vi "JH setpoint feedback off before point spectra.vi"() -> ()   [LabVIEW 2014]
uses:
  <userlib>/Nanonis Prog Interface V5/Nanonis Prog Interface.lvlib
panel:
  in  "spectroscopy feedback setpoint (V)":sgl=0.1 format="%_5p"
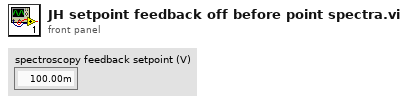
[diagram p1: front panel]
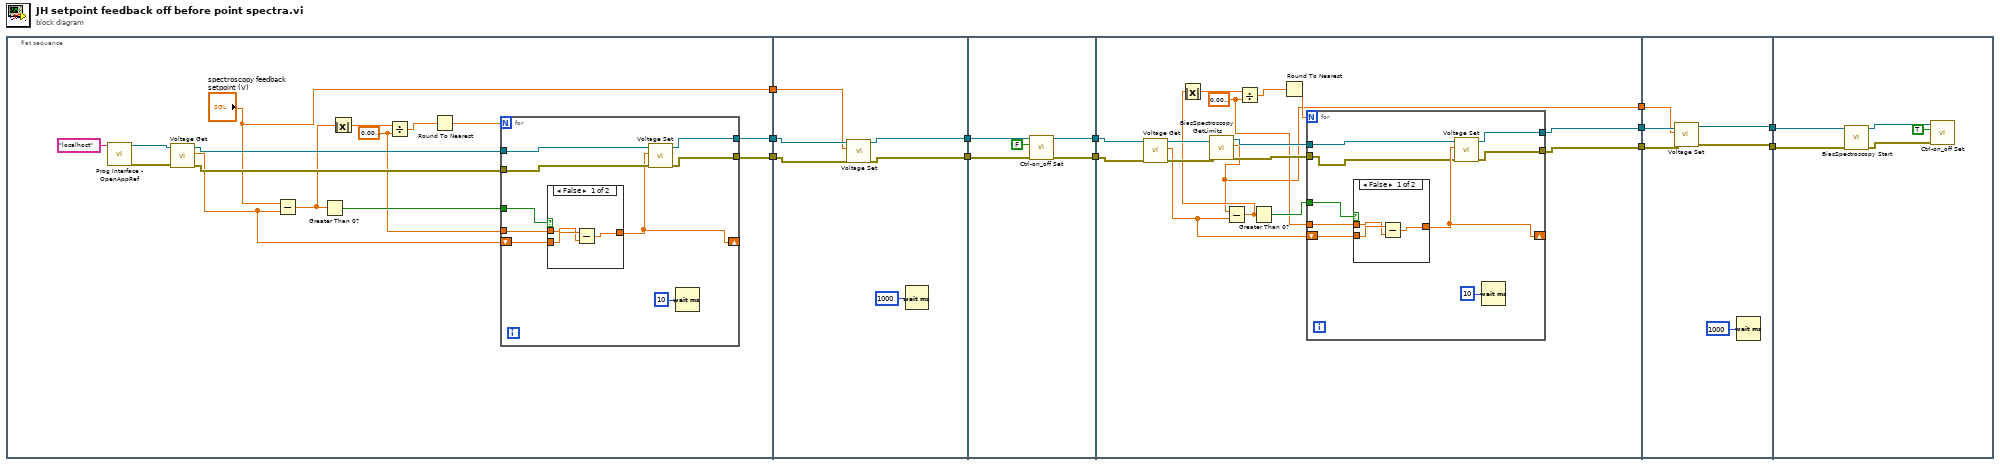
[diagram p0: block diagram]
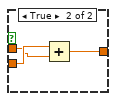
[diagram p2: hidden frame]
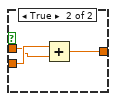
[diagram p3: hidden frame]
diagram:
  n1 = flat-sequence {
    tunnel: [w15] -> w4
    tunnel: [w14] -> w3
    tunnel: ["spectroscopy feedback setpoint (V)"] -> w2
    tunnel: [w45] -> w12
    tunnel: [w44] -> w11
    tunnel: w3 -> [w46]
    tunnel: w4 -> [w47]
    tunnel: w2 -> [w43]
    tunnel: w12 -> [w53]
    tunnel: w11 -> [w52]
    tunnel: [w50] -> w10
    tunnel: [w49] -> w9
    tunnel: w10 -> [w67]
    tunnel: w9 -> [w65]
    tunnel: [w56] -> w8
    tunnel: [w55] -> w6
    tunnel: [w54] -> w1
    tunnel: w8 -> [w89]
    tunnel: [w87] -> w7
    tunnel: w6 -> [w88]
    tunnel: [w86] -> w5
    tunnel: w1 -> [w85]
    tunnel: w7 -> [w95]
    tunnel: w5 -> [w94]
    frame #0 {
      w16 = sgl 0.01 ("y")
      n2 = call <userlib>:"Prog Interface - OpenAppRef.vi"("Machine name (local machine IP)"="localhost") -> ("Error out"=w25:errorcluster, "Application reference"=w26:refnum<vi>)  [unwired: 5 in]
      n3 = call <userlib>:"Voltage Get.vi"("error in (no error)"=w25, "Application ref in"=w26) -> ("error out"=w23:errorcluster, "Bias (V)"=w17:sgl, "Application ref out"=w24:refnum<vi>)  [unwired: 7 in]
      n4 = Subtract(x="spectroscopy feedback setpoint (V)", y=w17) -> (x-y=w21:sgl)
      n5 = Greater Than 0?(x=w21) -> (x > 0?=w22:bool)
      n6 = Absolute Value(x=w21) -> (abs(x)=w20:sgl)
      n7 = Divide(x=w20, y=w16) -> (x/y=w19:sgl)
      n8 = Round To Nearest(number=w19) -> (nearest integer value=w18:sgl)
      n9 = for {
        N: w18 -> [_]
        tunnel: w24 -> [w36]
        tunnel: w23 -> [w35]
        tunnel: w22 -> [w34]
        tunnel: w16 -> [w33]
        shift-right: [w31] -> _
        shift-left: w17 -> [w32]
        tunnel: [w29] -> w15
        tunnel: [w28] -> w14
        n10 = case shown="False" w34 {
          tunnel: w33 -> [w38 w41]
          tunnel: w32 -> [w39 w42]
          tunnel: [w37 w40] -> w31
          frame False {
            n11 = Subtract(x=w39, y=w38) -> (x-y=w37:sgl)
          }
          frame True {
            n12 = Add(x=w42, y=w41) -> (x+y=w40:sgl)
          }
        }
        n13 = call <userlib>:"Voltage Set.vi"("Error in (no error)"=w35, "Bias (V)"=w31, "Application ref in"=w36) -> ("Error out"=w28:errorcluster, "Application ref out"=w29:refnum<vi>)  [unwired: 7 in]
        n14 = Wait (ms)(milliseconds to wait=u32 10) -> ()  [unwired: 1 out]
      }
    }
    frame #1 {
      n15 = call <userlib>:"Voltage Set.vi"("Error in (no error)"=w46, "Bias (V)"=w43, "Application ref in"=w47) -> ("Error out"=w44:errorcluster, "Application ref out"=w45:refnum<vi>)  [unwired: 7 in]
      n16 = Wait (ms)(milliseconds to wait=u32 1000) -> ()  [unwired: 1 out]
    }
    frame #2 {
      n17 = call <userlib>:"Ctrl-on_off Set.vi"("error in (no error)"=w52, "Z Controller ON/OFF"=FALSE, "Application ref in"=w53) -> ("error out"=w49:errorcluster, "Application ref out"=w50:refnum<vi>)  [unwired: 7 in]
    }
    frame #3 {
      w57 = sgl 0.01 ("y")
      n18 = call <userlib>:"Voltage Get.vi"("error in (no error)"=w65, "Application ref in"=w67) -> ("error out"=w64:errorcluster, "Bias (V)"=w62:sgl, "Application ref out"=w66:refnum<vi>)  [unwired: 7 in]
      n19 = call <userlib>:"BiasSpectroscopy GetLimits.vi"("Error in (no error)"=w64, "Application ref in"=w66) -> ("Error out"=w68:errorcluster, "Start value (V)"=w54:sgl, "Application ref out"=w69:refnum<vi>)  [unwired: 4 in, 1 out]
      n20 = Subtract(x=w54, y=w62) -> (x-y=w58:sgl)
      n21 = Absolute Value(x=w58) -> (abs(x)=w61:sgl)
      n22 = Divide(x=w61, y=w57) -> (x/y=w60:sgl)
      n23 = Greater Than 0?(x=w58) -> (x > 0?=w63:bool)
      n24 = Round To Nearest(number=w60) -> (nearest integer value=w59:sgl)
      n25 = for {
        N: w59 -> [_]
        tunnel: w69 -> [w71]
        tunnel: w63 -> [w78]
        tunnel: w57 -> [w77]
        shift-right: [w75] -> _
        shift-left: w62 -> [w76]
        tunnel: [w73] -> w56
        tunnel: [w72] -> w55
        tunnel: w68 -> [w70]
        n26 = case shown="False" w78 {
          tunnel: w77 -> [w80 w83]
          tunnel: w76 -> [w81 w84]
          tunnel: [w79 w82] -> w75
          frame False {
            n27 = Subtract(x=w81, y=w80) -> (x-y=w79:sgl)
          }
          frame True {
            n28 = Add(x=w84, y=w83) -> (x+y=w82:sgl)
          }
        }
        n29 = call <userlib>:"Voltage Set.vi"("Error in (no error)"=w70, "Bias (V)"=w75, "Application ref in"=w71) -> ("Error out"=w72:errorcluster, "Application ref out"=w73:refnum<vi>)  [unwired: 7 in]
        n30 = Wait (ms)(milliseconds to wait=u32 10) -> ()  [unwired: 1 out]
      }
    }
    frame #4 {
      n31 = call <userlib>:"Voltage Set.vi"("Error in (no error)"=w88, "Bias (V)"=w85, "Application ref in"=w89) -> ("Error out"=w86:errorcluster, "Application ref out"=w87:refnum<vi>)  [unwired: 7 in]
      n32 = Wait (ms)(milliseconds to wait=u32 1000) -> ()  [unwired: 1 out]
    }
    frame #5 {
      n33 = call <userlib>:"BiasSpectroscopy Start.vi"("Application ref in"=w95, "Error in (no error)"=w94) -> ("Application ref out"=w93:refnum<vi>, "Error out"=w92:errorcluster)  [unwired: 9 in, 3 out]
      n34 = call <userlib>:"Ctrl-on_off Set.vi"("error in (no error)"=w92, "Z Controller ON/OFF"=TRUE, "Application ref in"=w93) -> ()  [unwired: 7 in, 2 out]
    }
  }
